vi "robot_dis.vi"() -> ()   [LabVIEW 2014]
uses:
  <vilib>/robotics/Controls/2D Rangefinder/NI_Robotics_2D Rangefinder.xctl
  <vilib>/Utility/error.llb/DialogType.ctl
  <vilib>/picture/3D Picture Control/Object/Create Object (drawable).vi
  <vilib>/picture/3D Picture Control/Object/Add Object (reference).vi
  <vilib>/picture/3D Picture Control/NI_3D Picture Control.lvlib
panel:
  out "布尔 3":bool=TRUE
  out "Lidar_two":i32
  out "StopChannelRecord":bool
  out "StartChannelRecord":bool
  out "布尔 2":bool
  in  "开始录像":bool
  in  "布尔":bool
  out "StartChannelRealPlay":bool
  in  "Lidar_data":cluster{"数组":dbl[], "数组 2":dbl[][]}
  out "Rangefinder Indicator":cluster{"angle":dbl[], "distance":dbl[][]}(xcontrol)
  out "扫描质量":u8
  out "Lidar_size":u16
  in  "distance":dbl[](array[numeric])
  in  "angle":dbl[](array[numeric])
  out "数值 2":u8 format="%x"
  out "x或y?":u8 format="%x"
  out "x = y?":bool
  out "无符号字节数组 2":u8[](array[numeric])
  out "动力电池":dbl(slide) scale=0.0..100.0
  out "控制电池":dbl(slide) scale=0.0..100.0 scale format="%.3f"
  in  "主要":refnum<k7>(container)
  in  "后摄像头":refnum<k7>(container)
  out "Login 2":i32
  out "前摄像头":bool
  out "后摄像头":bool
  out "Login":i32
  in  "前摄像头":refnum<k7>(container)
  in  "AUTO":bool
  in  "减速":bool
  in  "加速":bool
  in  "左":bool
  in  "右":bool
  in  "下":bool
  in  "上":bool
  in  "LED8":u8(slide) step=1 scale=0.0..100.0
  in  "LED7":u8(slide) step=1 scale=0.0..100.0
  in  "LED6":u8(slide) step=1 scale=0.0..100.0
  in  "LED5":u8(slide) step=1 scale=0.0..100.0
  in  "LED4":u8(slide) step=1 scale=0.0..100.0
  in  "LED3":u8(slide) step=1 scale=0.0..100.0
  in  "LED2":u8(slide) step=1 scale=0.0..100.0
  in  "LED1":u8(slide) step=1 scale=0.0..100.0
  in  "上下移动":dbl(slide) scale=-10.0..10.0
  in  "左右移动":dbl(slide) scale=-10.0..10.0
  in  "前后移动":dbl(slide) scale=-10.0..10.0
  in  "缩放":dbl(knob)=2.2771854734286614 scale=0.0..10.0
  out "小车方向":refnum<vi>(3d-picture)
  out "HEANDING":i32
  out "BANK":i32
  out "PITCH":i32
  in  "方向枚举":enum16{"停", "上", "下", "左", "右"}(ring)
  out "和":u8
  out "Car_lock":u8
  out "当前速度":u16
  out "当前方向":u8
  out "数据传输":bool
  in  "数据输入":string
  in  "QUIT":bool
  in  "WRITE":bool
  # "TETRAELC--机器人测试平台V0.1"
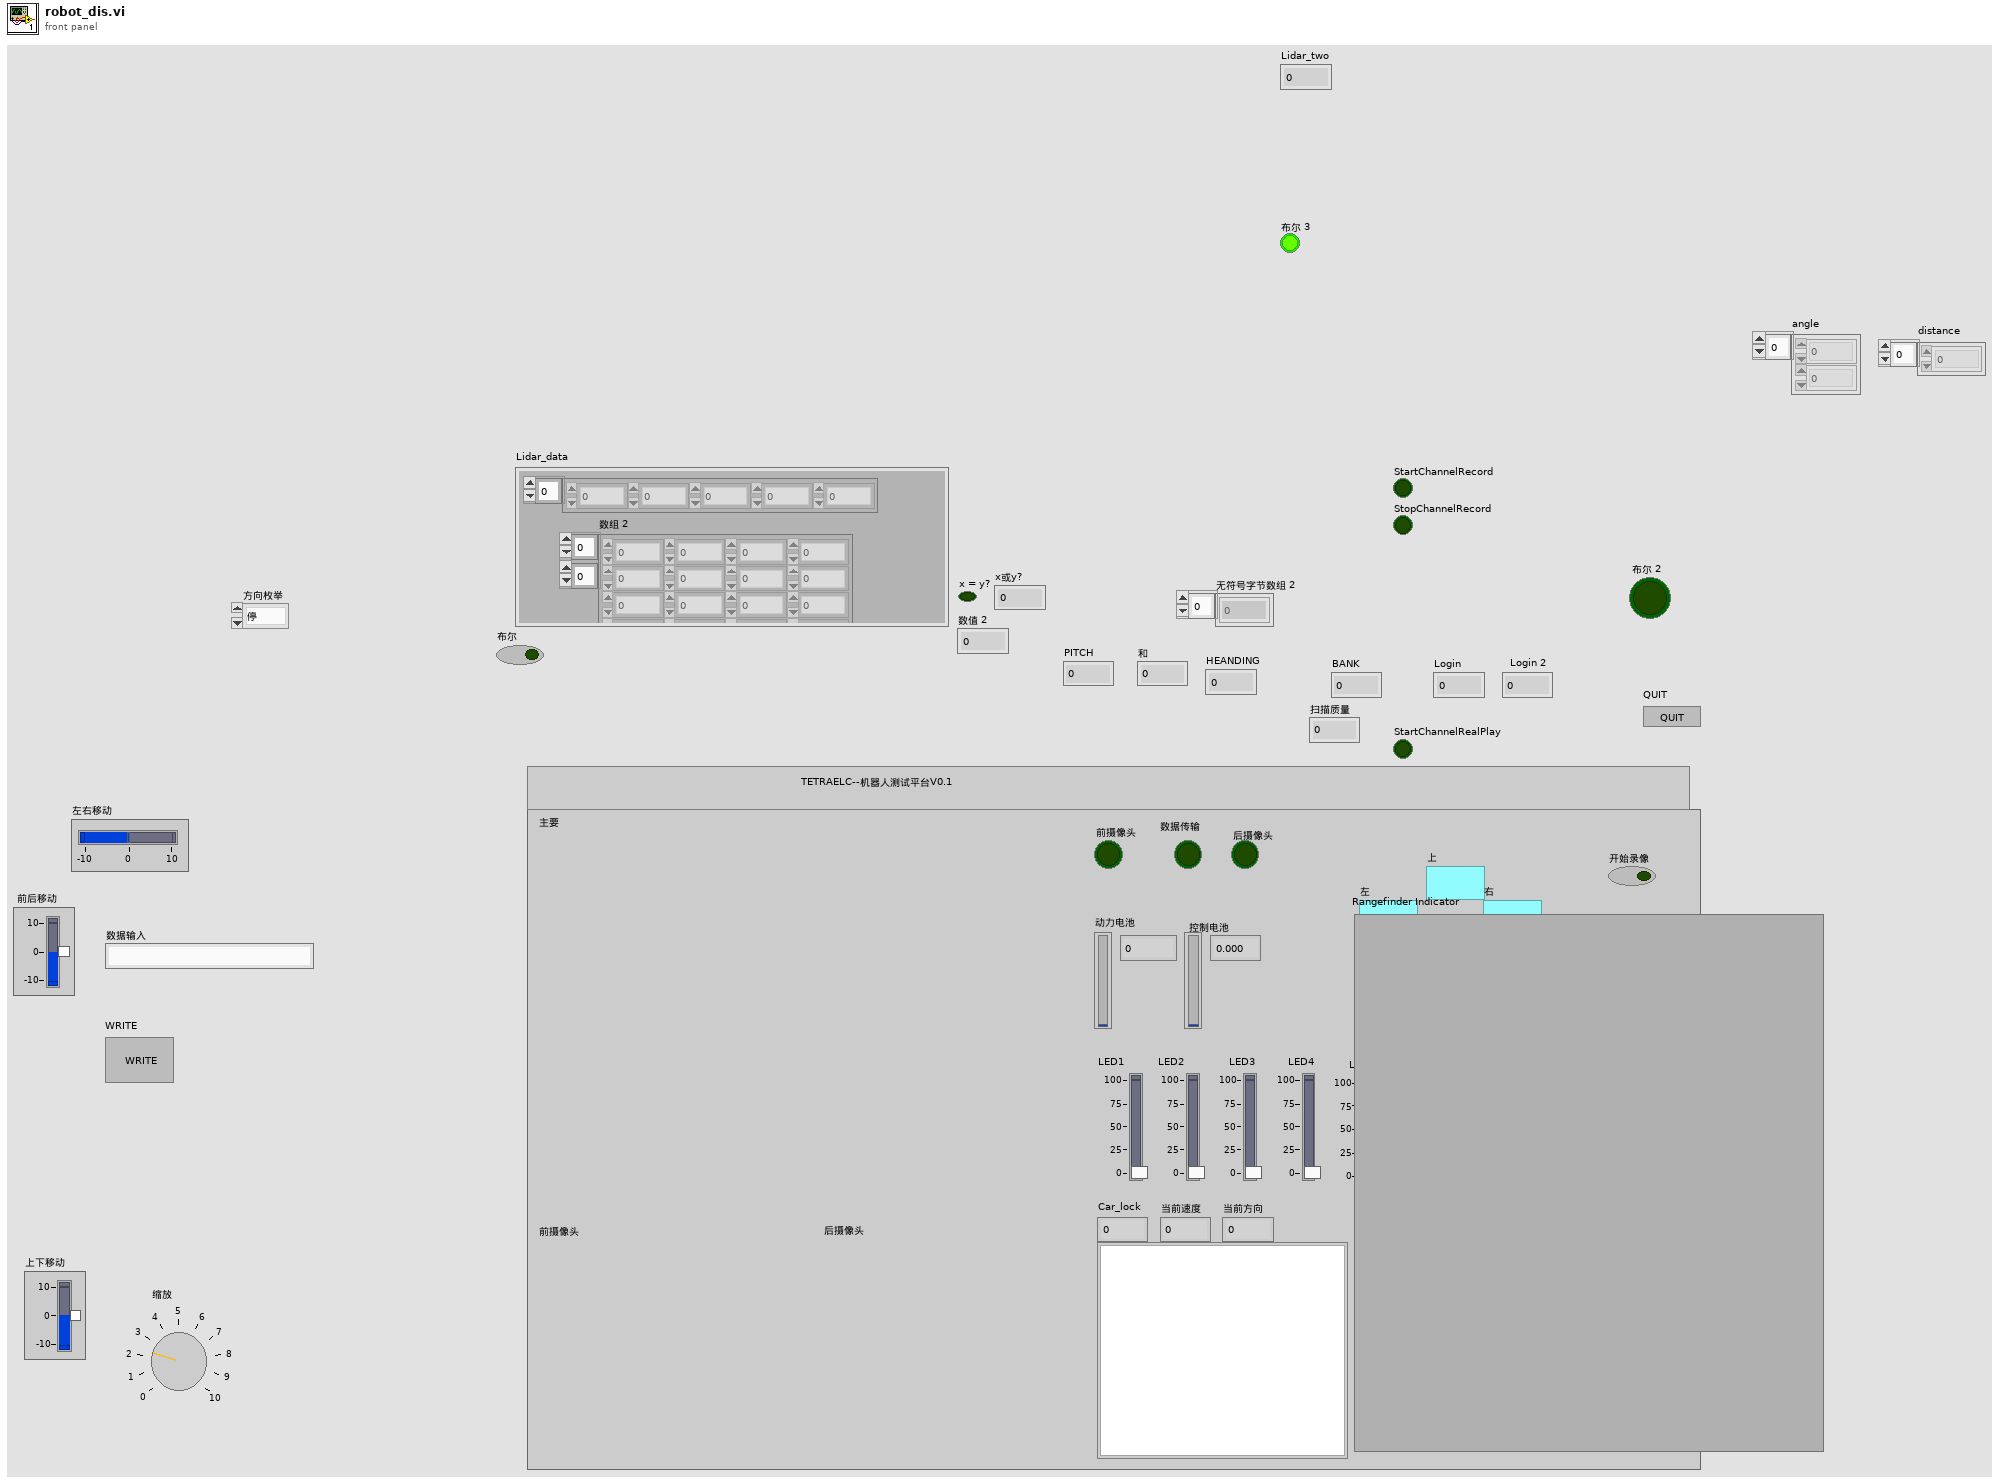
[diagram p1: front panel]
types:
  T1 = typedef "DialogType.ctl" = u16
  T2 = cluster{"PITCH":i32, "BANK":i32, "HEANDING":i32, "X":i32, "Y":i32, "Z":i32}
  T3 = cluster{"quality":u8, "angle":u16, "distance\n":u16}
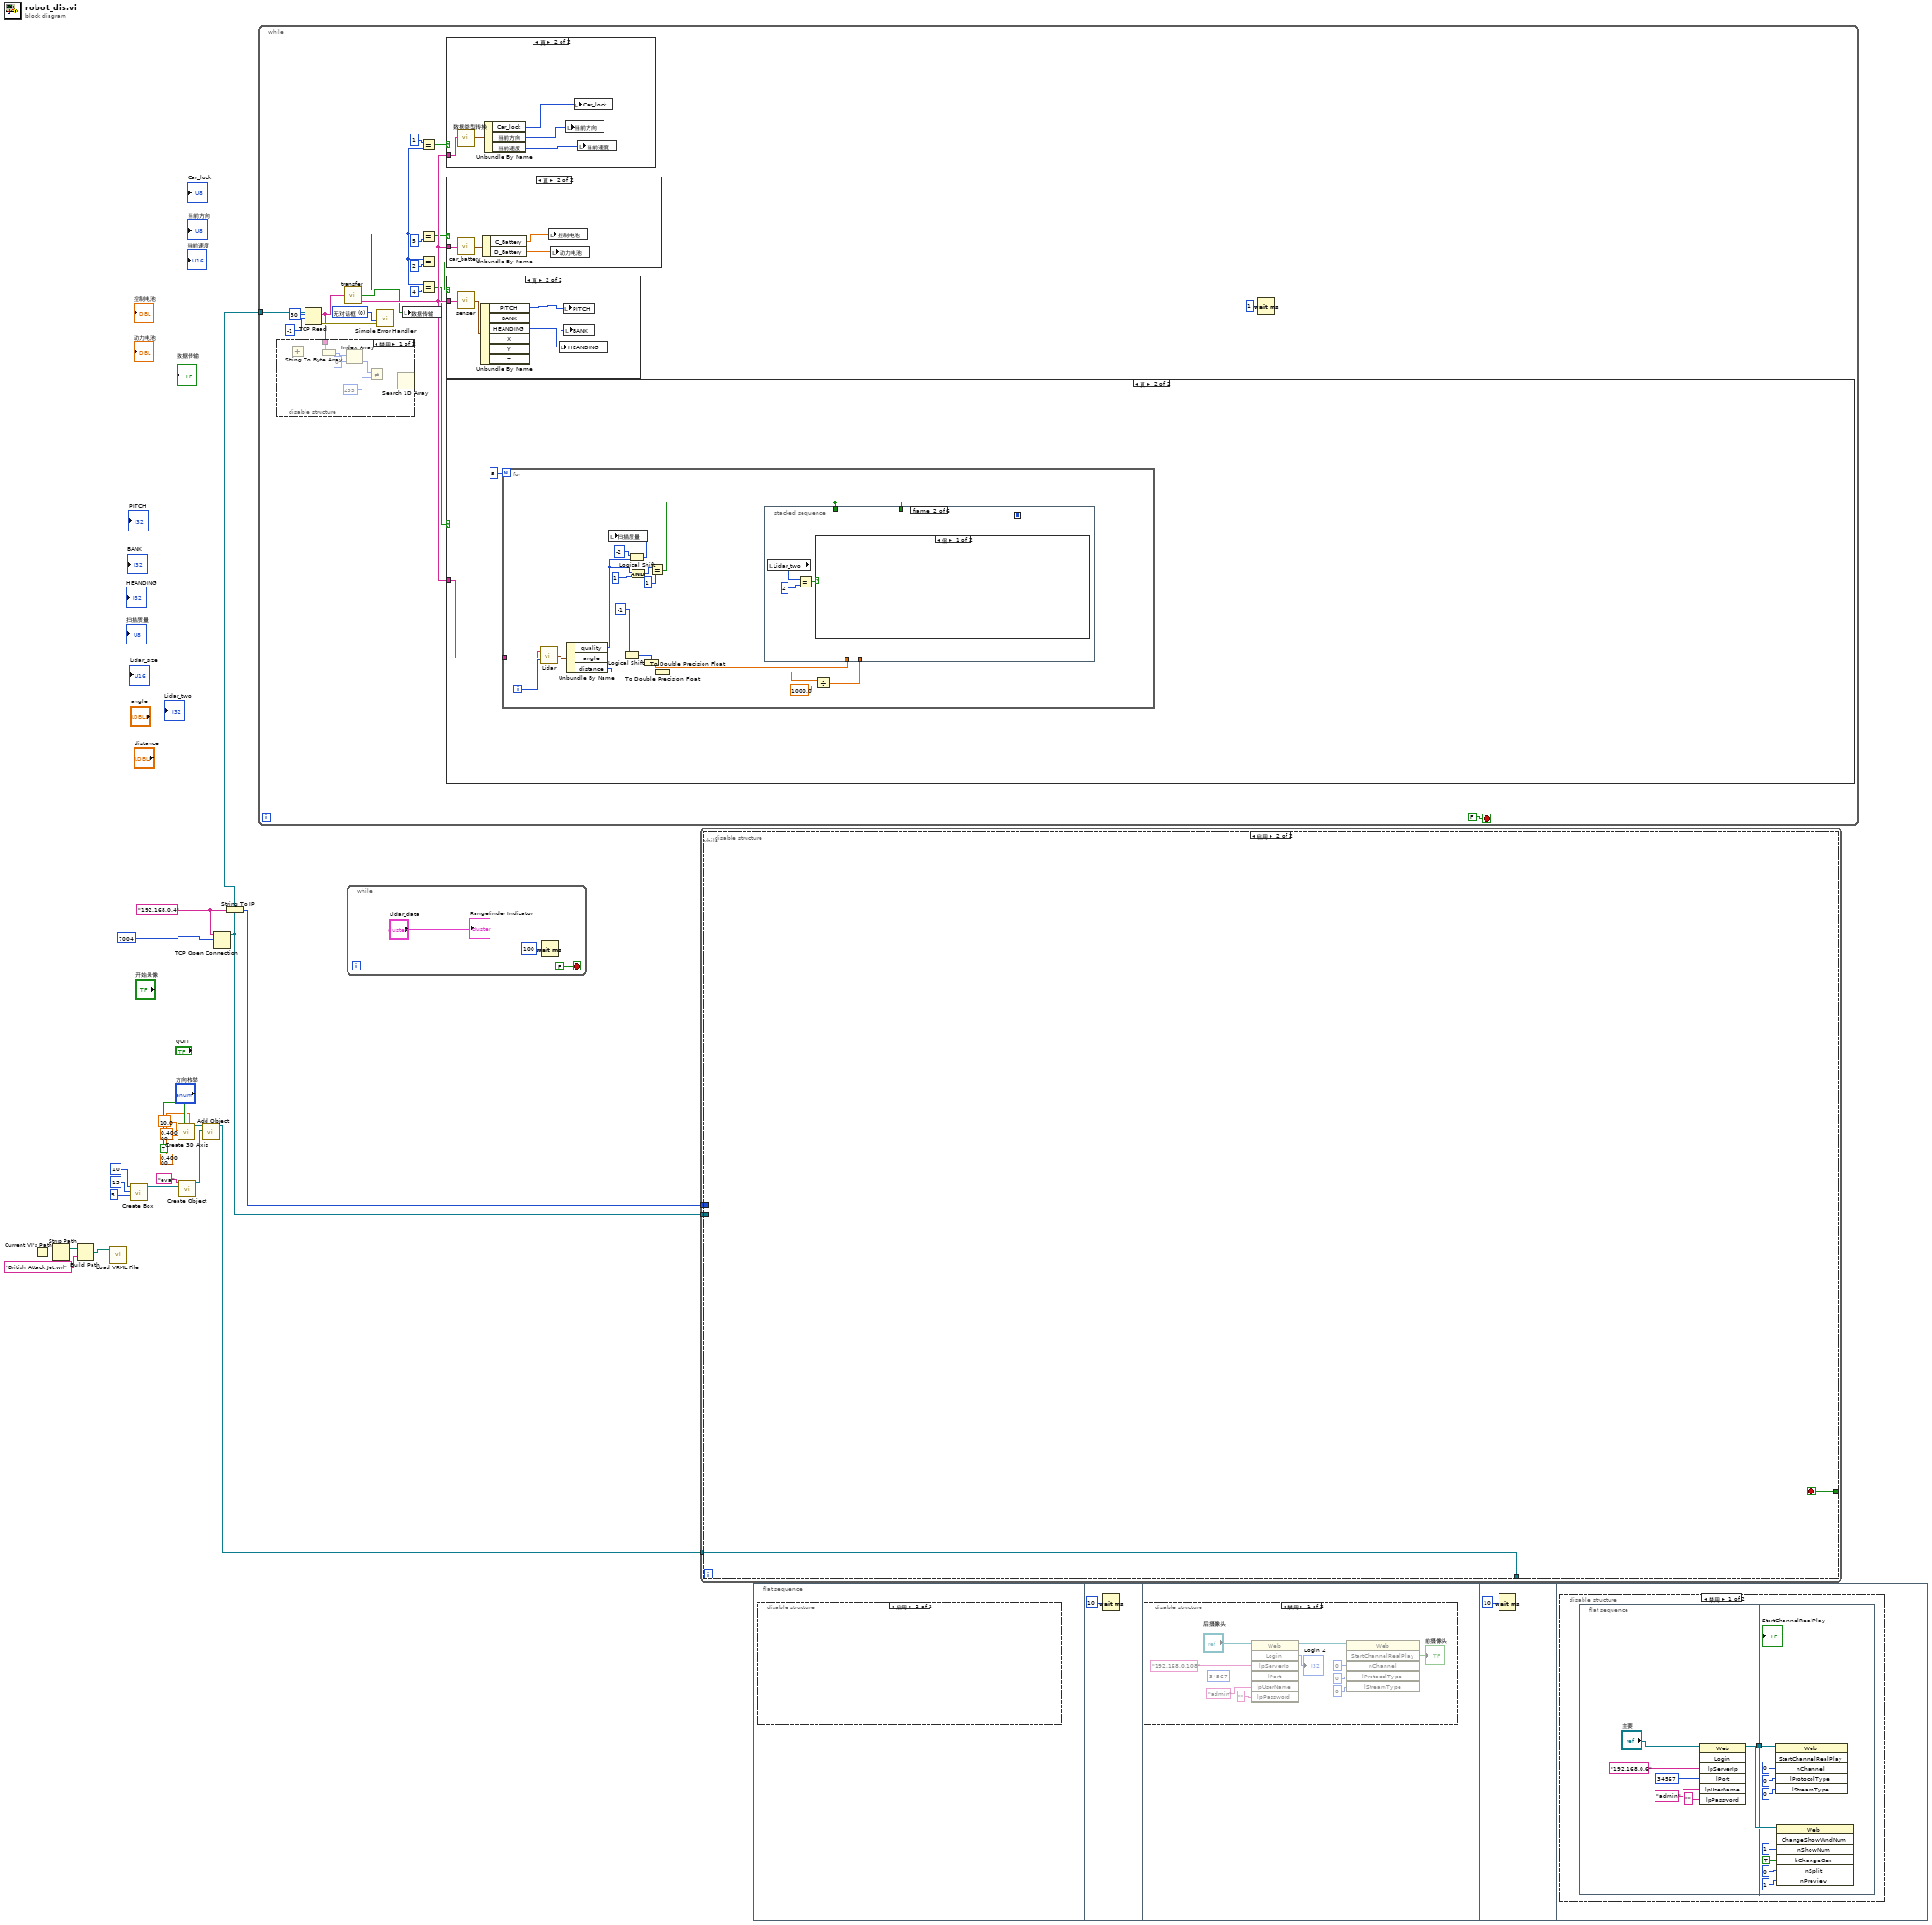
[diagram p0: block diagram]
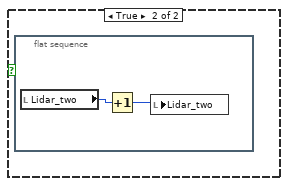
[diagram p5: hidden frame]
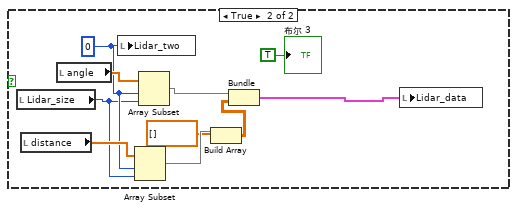
[diagram p6: hidden frame]
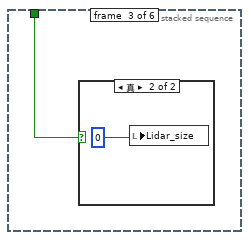
[diagram p7: hidden frame]
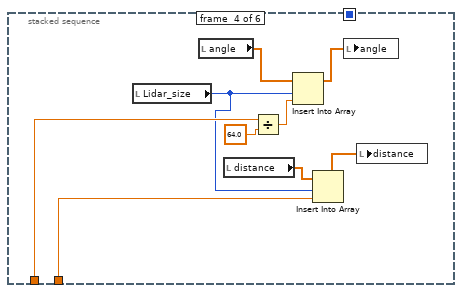
[diagram p9: hidden frame]
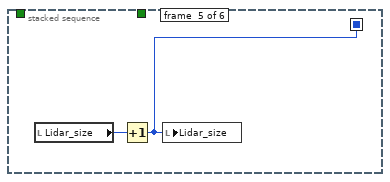
[diagram p10: hidden frame]
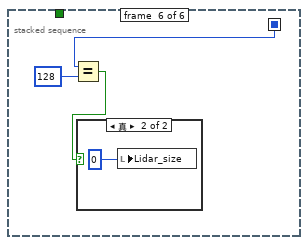
[diagram p11: hidden frame]
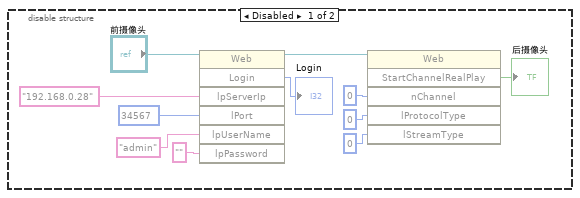
[diagram p16: hidden frame]
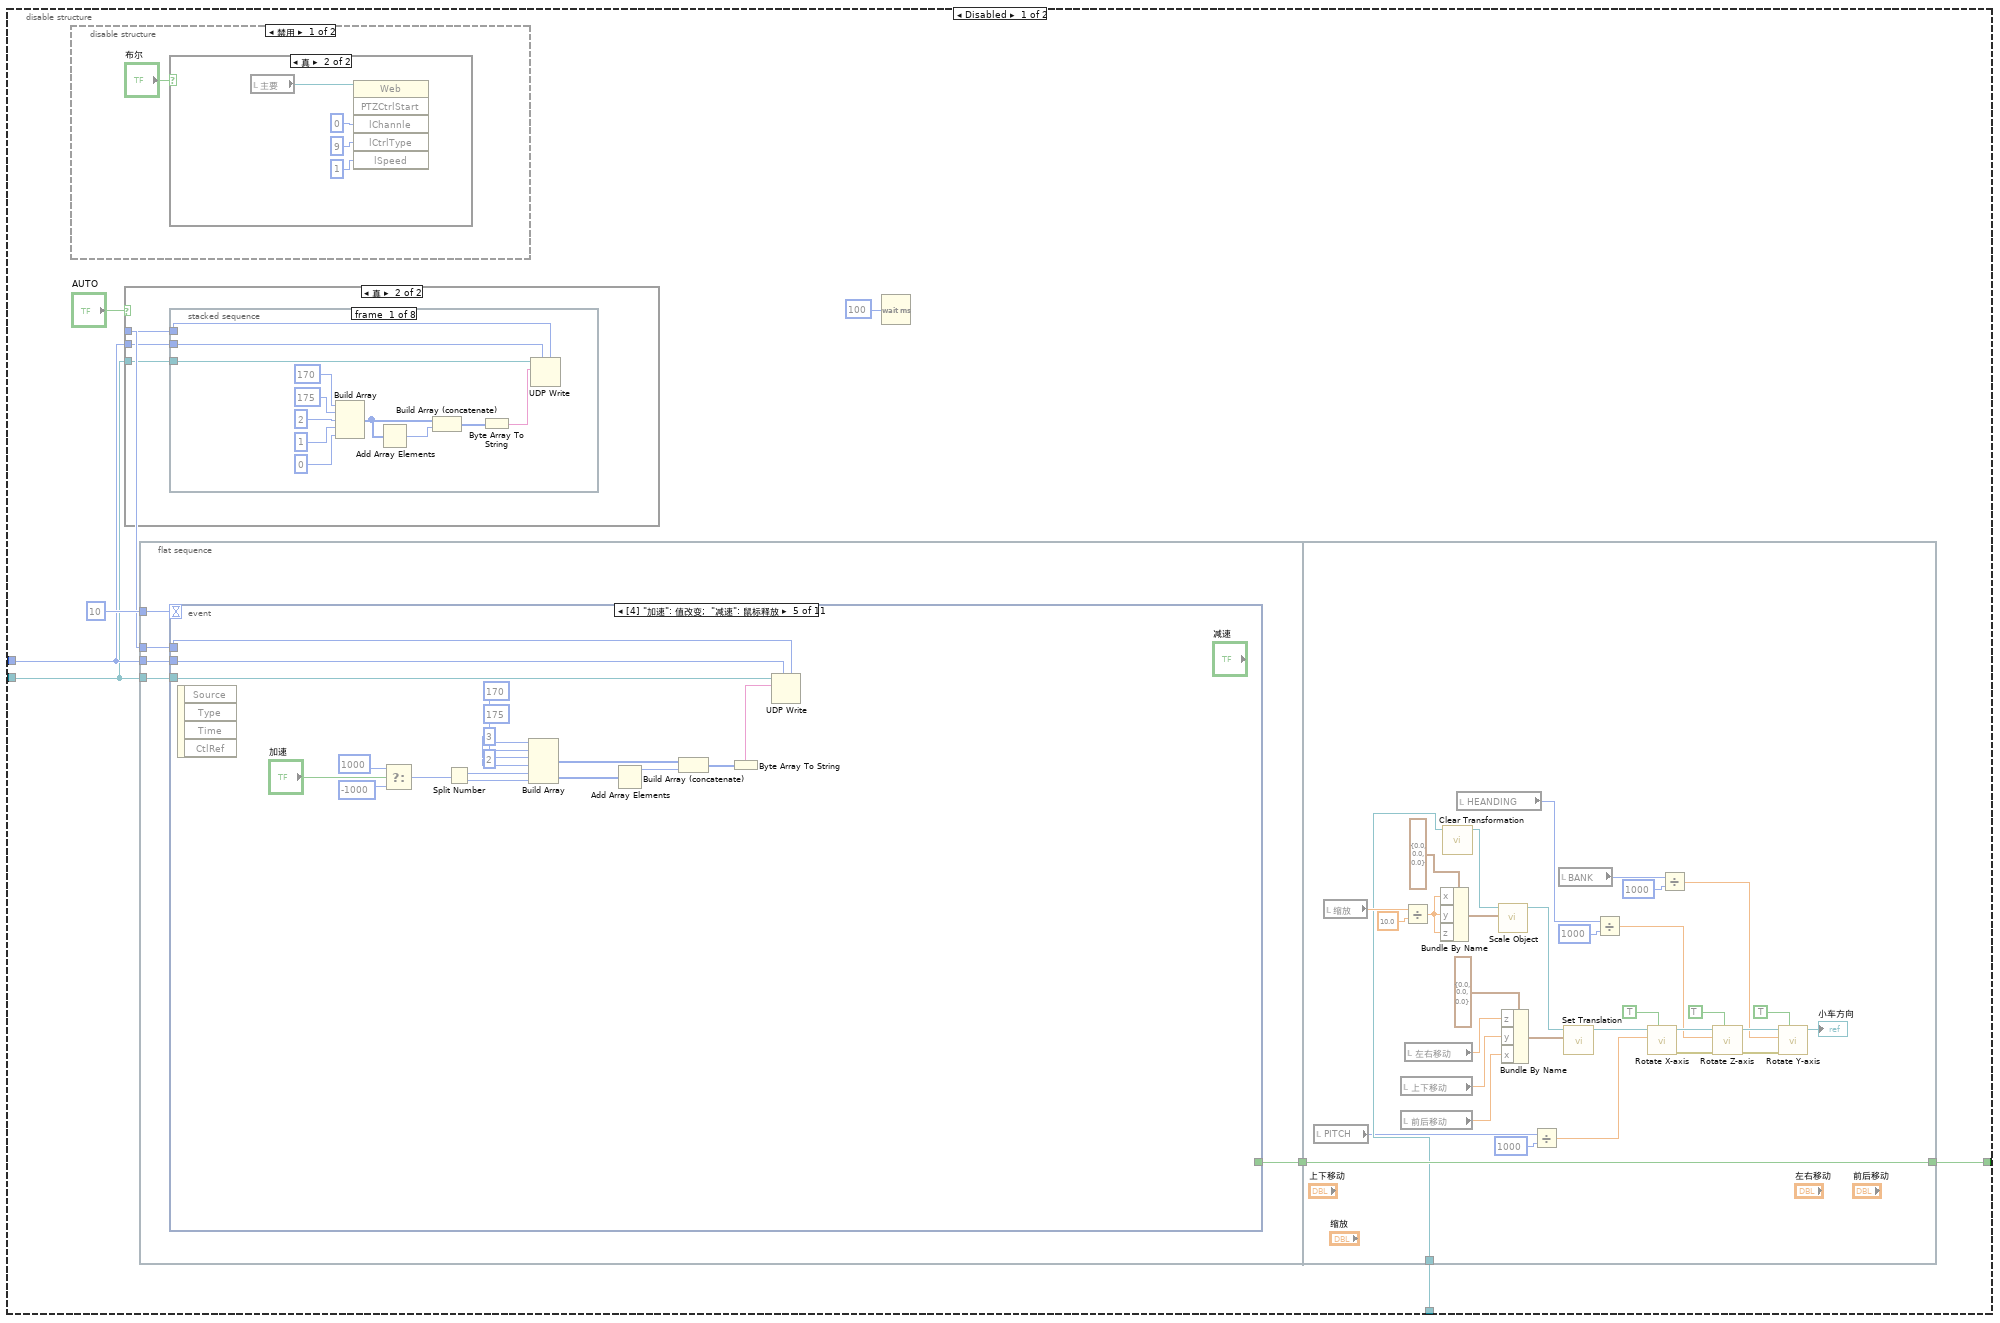
[diagram p19: hidden frame]
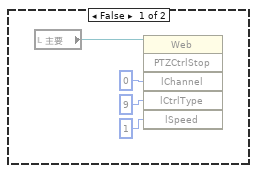
[diagram p20: hidden frame]
diagram:
  w1 = "192.168.0.4" ("目标主机")
  n1 = Current VI's Path() -> (path=w7:path)
  n2 = Strip Path(path=w7) -> (stripped path=w6:path)  [unwired: 1 out]
  n3 = Build Path(base path=w6, name or relative path="British Attack Jet.wrl" ("Name")) -> (appended path=w8:path)
  n4 = call <vilib>:"Load VRML File.vi"("Path"=w8) -> ()  [unwired: 9 in, 2 out]
  n5 = call <vilib>:"Create Box.vi"("Length Z"=5, "Length Y"=15, "Length X"=10) -> ("New Box Refnum"=w15:refnum<vi>)  [unwired: 7 in, 1 out]
  n6 = call <vilib>:"Create 3D Axis.vi"("Character Size"=sgl 0.4, "Axis label?"=TRUE, "Radius"=sgl 0.4, "Length"=sgl 10.0) -> ("New Object Refnum"=w10:refnum<vi>)  [unwired: 6 in, 1 out]
  n7 = call-poly <vilib>:"Create Object.vi"("Geometry"=w15, "Name"="eva") -> ("Scene:New Object"=w4:refnum<vi>)  [unwired: 8 in, 1 out]
  n8 = call-poly <vilib>:"Add Object.vi"("New Object In"=w4, "Scene Object In"=w10) -> ("Scene Object Out"=w9:refnum<vi>)  [unwired: 7 in, 2 out]
  n9 = TCP Open Connection(address=w1, remote port or service name=u16 7004 ("本地端口")) -> (connection ID=w2:refnum<k5>)  [unwired: 3 in, 1 out]
  n10 = String To IP(1:w1) -> (0:w20:u32)
  n11 = while {
    tunnel: w2 -> [w25]
    stop <- FALSE stop-if-true
    w28 = T1 0 items=["无对话框", "确定信息", "继续或停止信息", "确定信息＋警告", "继续/停止+警告"] ("type of dialog (OK msg:1)")
    n12 = TCP Read(connection ID=w25, bytes to read=30 ("读取的字节"), 9:-1 ("超时毫秒(25000)")) -> (data out=w22:string, error out=w23:errorcluster)  [unwired: 2 in, 1 out]
    n13 = disable-structure shown="禁用" {
      disable-tunnel: w22 -> [w44 _]
      frame Disabled {
        n14 = Add() -> ()  [unwired: 2 in, 1 out]
        n15 = String To Byte Array(string=w44) -> (unsigned byte array=w43:u8[])
        n16 = Index Array(array=w43, index=0 ("索引")) -> (element=w41:u8)
        n17 = Not Equal?(x=w41, y=u8 255 ("元素")) -> ()  [unwired: 1 out]
        n18 = Search 1D Array() -> ()  [unwired: 3 in, 1 out]
      }
      frame Enabled {
      }
    }
    n19 = call "transfer.vi"("输入"=w22) -> ("数值"=w35:u8, "布尔"=w27:bool, "输出"=w38:string)
    n20 = call <vilib>:"Simple Error Handler.vi"("type of dialog (OK msg:1)"=w28, "error in (no error)"=w23) -> ()  [unwired: 3 in, 5 out]
    n21 = local write "数据传输"(w27) -> ()
    n22 = Equal?(x=u8 1, y=w35) -> (x = y?=w30:bool)
    n23 = Equal?(x=w35, y=u8 5 ("x")) -> (x = y?=w34:bool)
    n24 = Equal?(x=w35, y=u8 2 ("x")) -> (x = y?=w32:bool)
    n25 = Equal?(x=w35, y=u8 4 ("x")) -> (x = y?=w37:bool)
    n26 = case shown="真" w30 {
      tunnel: w38 -> [_ w107]
      frame False {
      }
      frame True {
        n27 = call "数据类型转换.vi"("read buffer"=w107) -> ("输出簇"=w106:cluster{"Car_lock":u8, "当前方向":u8, "当前速度\n":u16})
        n28 = Unbundle By Name(w106) -> ("Car_lock"=w105:u8, "当前方向"=w104:u8, "当前速度"=w103:u16)
        n29 = local write "当前方向"(w104) -> ()
        n30 = local write "Car_lock"(w105) -> ()
        n31 = local write "当前速度"(w103) -> ()
      }
    }
    n32 = case shown="真" w34 {
      tunnel: w38 -> [_ w111]
      frame False {
      }
      frame True {
        n33 = call "car_battery.vi"("read buffer"=w111) -> ("输出簇"=w110:cluster{"C_Battery":dbl, "D_Battery\n":dbl})
        n34 = Unbundle By Name(w110) -> ("C_Battery"=w109:dbl, "D_Battery"=w108:dbl)
        n35 = local write "控制电池"(w109) -> ()
        n36 = local write "动力电池"(w108) -> ()
      }
    }
    n37 = case shown="真" w32 {
      tunnel: w38 -> [_ w102]
      frame False {
      }
      frame True {
        n38 = call "senser.vi"("read buffer"=w102) -> ("输出簇"=w101:T2)
        n39 = Unbundle By Name(w101) -> ("PITCH"=w100:i32, "BANK"=w99:i32, "HEANDING"=w98:i32)  [unwired: 3 out]
        n40 = local write "HEANDING"(w98) -> ()
        n41 = local write "PITCH"(w100) -> ()
        n42 = local write "BANK"(w99) -> ()
      }
    }
    n43 = case shown="真" w37 {
      tunnel: w38 -> [_ w46]
      frame False {
      }
      frame True {
        n44 = for {
          N: 5 -> [_]
          tunnel: w46 -> [w49]
          i -> [w47]
          n45 = call "Lidar.vi"("数值"=w47, "read buffer"=w49) -> ("输出簇"=w48:T3)
          n46 = Unbundle By Name(w48) -> ("quality"=w57:u8, "angle"=w61:u16, "distance"=w53:u16)
          n47 = Logical Shift(y=i16 -1, x=w61) -> (x << y=w60:u16)
          n48 = Logical Shift(y=i16 -2, x=w57) -> (x << y=w62:u8)
          n49 = local write "扫描质量"(w62) -> ()
          n50 = And(x=w57, y=u8 1) -> (x .and. y?=w56:u8)
          n51 = To Double Precision Float(number=w60) -> (double precision float=w58:dbl)
          n52 = Equal?(x=w56, y=u8 1) -> (x = y?=w54:bool)
          n53 = To Double Precision Float(number=w53) -> (double precision float=w52:dbl)
          n54 = Divide(x=w52, y=1000.0) -> (x/y=w50:dbl)
          n55 = stacked-sequence {
            seq-local: [_ _ _ _ w92 _] -> [_ _ _ _ _ w95]
            tunnel: w54 -> [w65 _ _ _ _ _]
            tunnel: w54 -> [_ _ w81 _ _ _]
            tunnel: w58 -> [_ _ _ w88 _ _]
            tunnel: w50 -> [_ _ _ w83 _ _]
            frame #0 {
              n56 = case shown="假" w65 {
                frame False {
                }
                frame True {
                  n57 = flat-sequence {
                    frame #0 {
                      n58 = local read "Lidar_two"() -> (w67:i32)
                      n59 = Increment(x=w67) -> (x+1=w66:i32)
                      n60 = local write "Lidar_two"(w66) -> ()
                    }
                  }
                }
              }
            }
            frame #1 {
              n61 = local read "Lidar_two"() -> (w70:i32)
              n62 = Equal?(x=w70, y=2) -> (x = y?=w68:bool)
              n63 = case shown="假" w68 {
                frame False {
                }
                frame True {
                  w78 = 0 ("Lidar_two")
                  n64 = local read "Lidar_size"() -> (w77:u16)
                  n65 = local read "distance"() -> (w79:dbl[])
                  n66 = local read "angle"() -> (w80:dbl[])
                  n67 = local write "Lidar_two"(w78) -> ()
                  n68 = Array Subset(array=w79, index=w78, length=w77) -> (w76:dbl[])
                  n69 = Array Subset(array=w80, index=w78, length=w77) -> (w74:dbl[])
                  n70 = Build Array(w76, dbl[] [] ("元素")) -> (w73:dbl[][])
                  n71 = Bundle(w74, w73) -> (w71:cluster{dbl[], dbl[][]})  [unwired: 1 in]
                  n72 = local write "Lidar_data"(w71) -> ()
                  "布尔 3" <- TRUE
                }
              }
            }
            frame #2 {
              n73 = case shown="真" w81 {
                frame False {
                }
                frame True {
                  n74 = local write "Lidar_size"(u8 0 ("Lidar_size")) -> ()
                }
              }
            }
            frame #3 {
              n75 = local read "Lidar_size"() -> (w84:u16)
              n76 = local read "angle"() -> (w91:dbl[])
              n77 = local read "distance"() -> (w85:dbl[])
              n78 = Divide(x=w88, y=64.0) -> (x/y=w87:dbl)
              n79 = Insert Into Array(array=w91, index=w84, new element=w87) -> (w90:dbl[])
              n80 = Insert Into Array(array=w85, index=w84, new element=w83) -> (w86:dbl[])
              n81 = local write "angle"(w90) -> ()
              n82 = local write "distance"(w86) -> ()
            }
            frame #4 {
              n83 = local read "Lidar_size"() -> (w93:u16)
              n84 = Increment(x=w93) -> (x+1=w92:u16)
              n85 = local write "Lidar_size"(w92) -> ()
            }
            frame #5 {
              n86 = Equal?(x=w95, y=u16 128) -> (x = y?=w94:bool)
              n87 = case shown="真" w94 {
                frame False {
                }
                frame True {
                  n88 = local write "Lidar_size"(u16 0 ("Lidar_size")) -> ()
                }
              }
            }
          }
        }
      }
    }
    n89 = Wait (ms)(milliseconds to wait=u32 1 ("等待时间（毫秒）")) -> ()  [unwired: 1 out]
  }
  n90 = while {
    stop <- FALSE stop-if-true
    n91 = Wait (ms)(milliseconds to wait=u32 100 ("等待时间（毫秒）")) -> ()  [unwired: 1 out]
    "Rangefinder Indicator" <- "Lidar_data"
  }
  n92 = while {
    tunnel: w2 -> [w115]
    tunnel: w20 -> [w116]
    tunnel: w9 -> [w117]
    stop <- w118 stop-if-true
    n93 = disable-structure shown="启用" {
      disable-tunnel: [w126 _] -> w118
      disable-tunnel: w117 -> [w124 _]
      disable-tunnel: w116 -> [w122 _]
      disable-tunnel: w115 -> [w121 _]
      frame Disabled {
        n94 = disable-structure shown="禁用" {
          frame Disabled {
            n95 = case shown="真" "布尔" {
              frame False {
                n96 = local read "主要"() -> (w132:refnum<k7>)
                n97 = invoke class="Web" method="PTZCtrlStop"(reference=w132, "lChannel"=0, "lCtrlType"=9, "lSpeed"=1) -> ()  [unwired: 2 in, 6 out]
              }
              frame True {
                n98 = local read "主要"() -> (w136:refnum<k7>)
                n99 = invoke class="Web" method="PTZCtrlStart"(reference=w136, "lChannle"=0, "lCtrlType"=9, "lSpeed"=1) -> ()  [unwired: 2 in, 6 out]
              }
            }
          }
          frame Enabled {
          }
        }
        n100 = case shown="真" "AUTO" {
          tunnel: [_ w139] -> w123
          tunnel: w122 -> [_ w138]
          tunnel: w121 -> [_ w137]
          frame False {
          }
          frame True {
            n101 = stacked-sequence {
              tunnel: w139 -> [w142 _ w153 _ w167 _ w180 _]
              tunnel: w138 -> [w141 _ w154 _ w168 _ w181 _]
              tunnel: w137 -> [w140 _ w155 _ w169 _ w179 _]
              frame #0 {
                n102 = Build Array(u8 170 ("元素"), u8 175 ("元素"), u8 2 ("元素"), u8 1 ("元素"), u8 0 ("元素")) -> (w146:u8[])
                n103 = Add Array Elements(numeric array=w146) -> (sum=w145:u8)
                n104 = Build Array (concatenate)(w146, w145) -> (w144:u8[])
                n105 = Byte Array To String(unsigned byte array=w144) -> (string=w151:string)
                n106 = UDP Write(address=w141, port or service name=w142, connection ID=w140, data in=w151) -> ()  [unwired: 2 in, 2 out]
              }
              frame #1 {
                n107 = Wait (ms)(milliseconds to wait=u32 3000 ("等待时间（毫秒）")) -> ()  [unwired: 1 out]
              }
              frame #2 {
                n108 = Build Array(u8 170 ("元素"), u8 175 ("元素"), u8 2 ("元素"), u8 1 ("元素"), u8 8 ("元素")) -> (w159:u8[])
                n109 = Add Array Elements(numeric array=w159) -> (sum=w158:u8)
                n110 = Build Array (concatenate)(w159, w158) -> (w157:u8[])
                n111 = Byte Array To String(unsigned byte array=w157) -> (string=w164:string)
                n112 = UDP Write(address=w154, port or service name=w153, connection ID=w155, data in=w164) -> ()  [unwired: 2 in, 2 out]
              }
              frame #3 {
                n113 = Wait (ms)(milliseconds to wait=u32 1000 ("等待时间（毫秒）")) -> ()  [unwired: 1 out]
              }
              frame #4 {
                n114 = Build Array(u8 170 ("元素"), u8 175 ("元素"), u8 2 ("元素"), u8 1 ("元素"), u8 1 ("元素")) -> (w173:u8[])
                n115 = Add Array Elements(numeric array=w173) -> (sum=w172:u8)
                n116 = Build Array (concatenate)(w173, w172) -> (w171:u8[])
                n117 = Byte Array To String(unsigned byte array=w171) -> (string=w177:string)
                n118 = UDP Write(address=w168, port or service name=w167, connection ID=w169, data in=w177) -> ()  [unwired: 2 in, 2 out]
              }
              frame #5 {
                n119 = Wait (ms)(milliseconds to wait=u32 3000 ("等待时间（毫秒）")) -> ()  [unwired: 1 out]
              }
              frame #6 {
                n120 = Build Array(u8 170 ("元素"), u8 175 ("元素"), u8 2 ("元素"), u8 1 ("元素"), u8 8 ("元素")) -> (w185:u8[])
                n121 = Add Array Elements(numeric array=w185) -> (sum=w184:u8)
                n122 = Build Array (concatenate)(w185, w184) -> (w183:u8[])
                n123 = Byte Array To String(unsigned byte array=w183) -> (string=w190:string)
                n124 = UDP Write(address=w181, port or service name=w180, connection ID=w179, data in=w190) -> ()  [unwired: 2 in, 2 out]
              }
              frame #7 {
                n125 = Wait (ms)(milliseconds to wait=u32 1000 ("等待时间（毫秒）")) -> ()  [unwired: 1 out]
              }
            }
          }
        }
        n126 = flat-sequence {
          tunnel: [w196] -> w127
          tunnel: 10 -> [w195]
          tunnel: w121 -> [w194]
          tunnel: w122 -> [w193]
          tunnel: w123 -> [w192]
          tunnel: [w415] -> w126
          tunnel: w127 -> [w415]
          tunnel: w124 -> [w389]
          frame #0 {
            n127 = event shown="[4] \"加速\": 值改变;  \"减速\": 鼠标释放" {
              selector: _ -> [_ _ _ _ _ _ _ _ _ _ _]
              dyn-events: _ -> [_ _ _ _ _ _ _ _ _ _ _]
              timeout: w195 -> [_ _ _ _ _ _ _ _ _ _ _]
              tunnel: [_ _ _ _ _ _ _ _ _ _ TRUE] -> w196
              tunnel: w194 -> [_ _ _ w259 w276 w296 w309 w331 w353 w378 w382]
              tunnel: w193 -> [_ _ _ w260 w277 w297 w310 w332 w354 w377 _]
              tunnel: w192 -> [_ _ _ w261 w278 w298 w311 w333 w355 w376 _]
              event Timeout {
                n128 = event-data() -> ()  [unwired: 1 in, 1 out]
                n129 = disable-structure shown="启用" {
                  disable-tunnel: _ -> [w213 _]
                  frame Disabled {
                    n130 = String Subset(string=w213, offset (0)=0 ("长度（剩余）"), length (rest)=100 ("长度（剩余）")) -> (substring=w223:string)
                    n131 = String To Byte Array(string=w223) -> (unsigned byte array=w210:u8[])
                    "无符号字节数组 2" <- w210
                    n132 = Index Array(array=w210, index #1=0 ("索引"), index #2=1 ("索引")) -> (element #1=w201:u8, element #2=w200:u8)
                    n133 = for {
                      N: 83 -> [_]
                      tunnel: w210 -> [w230]
                      shift-right: [w225] -> w199
                      shift-left: _ -> [w224]
                      i -> [w229]
                      n134 = Add(x=2, y=w229) -> (x+y=w227:i32)
                      n135 = Index Array(array=w230, index=w227) -> (element=w226:u8)
                      n136 = Exclusive Or(1:w224, 2:w226) -> (0:w225:u8)
                    }
                    "数值 2" <- w199
                    n137 = And(x=w200, y=u8 15) -> (x .and. y?=w203:u8)
                    n138 = Logical Shift(y=i16 -4, x=w201) -> (x << y=w216:u8)
                    n139 = Logical Shift(y=i16 -4, x=w200) -> (x << y=w214:u8)
                    n140 = Equal?(x=w214, y=u8 5) -> (x = y?=w211:bool)
                    n141 = Logical Shift(y=i16 4, x=w203) -> (x << y=w205:u8)
                    n142 = And(x=w201, y=u8 15) -> (x .and. y?=w204:u8)
                    n143 = Equal?(x=w216, y=u8 10) -> (x = y?=w212:bool)
                    n144 = And(x=w212, y=w211) -> (x .and. y?=w197:bool)
                    n145 = Or(x=w205, y=w204) -> (x .or. y?=w198:u8)
                    "x或y?" <- w198
                    n146 = case shown="真" w197 {
                      frame False {
                      }
                      frame True {
                        n147 = while {
                          stop <- FALSE stop-if-true
                        }
                        n148 = local read item#-1() -> (w232)
                        n149 = Increment(x=w232) -> (x+1=w231:dbl)
                        n150 = local write item#-1(w231) -> ()
                      }
                    }
                    n151 = Equal?(x=w198, y=w199) -> ()  [unwired: 1 out]
                  }
                  frame Enabled {
                  }
                }
              }
              event "Lidar_two": Value Change {
                n152 = event-data() -> ()  [unwired: 1 in, 6 out]
                n153 = disable-structure shown="禁用" {
                  frame Disabled {
                    n154 = local read "Lidar_two"() -> (w236:i32)
                    n155 = Equal?(x=w236, y=2) -> (x = y?=w234:bool)
                    n156 = case shown="真" w234 {
                      frame False {
                      }
                      frame True {
                      }
                    }
                  }
                  frame Enabled {
                  }
                }
              }
              event "开始录像": Value Change {
                n157 = event-data() -> ()  [unwired: 1 in, 6 out]
                n158 = local read "开始录像"() -> (w238:bool)
                n159 = local read "主要"() -> (w239:refnum<k7>)
                n160 = case shown="真" w238 {
                  tunnel: w239 -> [w243 w248]
                  tunnel: [FALSE ("布尔 2") TRUE ("布尔 2")] -> w237
                  frame False {
                    n161 = invoke class="Web" method="StopChannelRecord"(reference=w243, "nChannel"=0) -> ("StopChannelRecord"=→"StopChannelRecord":bool)  [unwired: 2 in, 3 out]
                  }
                  frame True {
                    n162 = invoke class="Web" method="StartChannelRecord"(reference=w248, "nChannel"=0, "lpSaveFile"="D:\\record", "nType"=0) -> ("StartChannelRecord"=→"StartChannelRecord":bool)  [unwired: 2 in, 5 out]
                  }
                }
                "布尔 2" <- w237
              }
              event "LED1", "LED2", "LED3", "LED4", "LED5", "LED6", "LED7", "LED8": Value Change {
                n163 = event-data() -> ()  [unwired: 1 in, 6 out]
                n164 = Build Array(u8 170 ("元素"), u8 175 ("元素"), u8 4 ("元素"), u8 8 ("元素"), "LED1", "LED2", "LED3", "LED4", "LED5", "LED6", "LED7", "LED8") -> (w265:u8[])
                n165 = Add Array Elements(numeric array=w265) -> (sum=w264:u8)
                "和" <- w264
                n166 = Build Array (concatenate)(w265, w264) -> (w263:u8[])
                n167 = Byte Array To String(unsigned byte array=w263) -> (string=w258:string)
                n168 = UDP Write(address=w260, port or service name=w261, connection ID=w259, data in=w258, 9:250 ("超时毫秒(25000)")) -> ()  [unwired: 1 in, 2 out]
              }
              event "加速": Value Change; "减速": Mouse Up {
                n169 = event-data() -> ()  [unwired: 1 in, 4 out]
                n170 = Select(t=i16 1000 ("x"), s="加速", f=i16 -1000) -> (s? t:f=w271:i16)
                n171 = Split Number(x=w271) -> (hi(x)=w275:u8, lo(x)=w274:u8)
                n172 = Build Array(u8 170 ("元素"), u8 175 ("元素"), u8 3 ("元素"), u8 2 ("元素"), w275, w274) -> (w281:u8[])
                n173 = Add Array Elements(numeric array=w281) -> (sum=w280:u8)
                n174 = Build Array (concatenate)(w281, w280) -> (w279:u8[])
                n175 = Byte Array To String(unsigned byte array=w279) -> (string=w286:string)
                n176 = UDP Write(address=w277, port or service name=w278, connection ID=w276, data in=w286) -> ()  [unwired: 2 in, 2 out]
              }
              event "上": Value Change {
                n177 = event-data() -> ()  [unwired: 1 in, 6 out]
                n178 = flat-sequence {
                  tunnel: [w303] -> w287
                  frame #0 {
                    n179 = case shown="真" "上" {
                      frame False {
                        n180 = local write "方向枚举"(enum16{"停", "上", "下", "左", "右"}."停") -> ()
                      }
                      frame True {
                        n181 = local write "方向枚举"(enum16{"停", "上", "下", "左", "右"}."上") -> ()
                      }
                    }
                  }
                  frame #1 {
                    n182 = local read "方向枚举"() -> (w302:enum16{"停", "上", "下", "左", "右"})
                    n183 = case shown="\"上\", 默认" w302 {
                      tunnel: [u8 0 ("元素") u8 1 ("元素") u8 2 ("元素") u8 3 ("元素") u8 8 ("元素")] -> w303
                      frame "上", Default {
                      }
                      frame "下" {
                      }
                      frame "左" {
                      }
                      frame "右" {
                      }
                      frame "停" {
                      }
                    }
                  }
                }
                n184 = Build Array(u8 170 ("元素"), u8 175 ("元素"), u8 2 ("元素"), u8 1 ("元素"), w287) -> (w290:u8[])
                n185 = Add Array Elements(numeric array=w290) -> (sum=w289:u8)
                n186 = Build Array (concatenate)(w290, w289) -> (w288:u8[])
                n187 = Byte Array To String(unsigned byte array=w288) -> (string=w295:string)
                n188 = UDP Write(address=w297, port or service name=w298, connection ID=w296, data in=w295) -> ()  [unwired: 2 in, 2 out]
              }
              event "下": Value Change {
                n189 = event-data() -> ()  [unwired: 1 in, 6 out]
                n190 = flat-sequence {
                  tunnel: [w325] -> w312
                  frame #0 {
                    n191 = case shown="真" "下" {
                      frame False {
                        n192 = local write "方向枚举"(enum16{"停", "上", "下", "左", "右"}."停") -> ()
                      }
                      frame True {
                        n193 = local write "方向枚举"(enum16{"停", "上", "下", "左", "右"}."下") -> ()
                      }
                    }
                  }
                  frame #1 {
                    n194 = local read "方向枚举"() -> (w324:enum16{"停", "上", "下", "左", "右"})
                    n195 = case shown="\"上\", 默认" w324 {
                      tunnel: [u8 0 ("元素") u8 1 ("元素") u8 2 ("元素") u8 3 ("元素") u8 8 ("元素")] -> w325
                      frame "上", Default {
                      }
                      frame "下" {
                      }
                      frame "左" {
                      }
                      frame "右" {
                      }
                      frame "停" {
                      }
                    }
                  }
                }
                n196 = Build Array(u8 170 ("元素"), u8 175 ("元素"), u8 2 ("元素"), u8 1 ("元素"), w312) -> (w315:u8[])
                n197 = Add Array Elements(numeric array=w315) -> (sum=w314:u8)
                n198 = Build Array (concatenate)(w315, w314) -> (w313:u8[])
                n199 = Byte Array To String(unsigned byte array=w313) -> (string=w320:string)
                n200 = UDP Write(address=w310, port or service name=w311, connection ID=w309, data in=w320) -> ()  [unwired: 2 in, 2 out]
              }
              event "左": Value Change {
                n201 = event-data() -> ()  [unwired: 1 in, 6 out]
                n202 = flat-sequence {
                  tunnel: [w347] -> w334
                  frame #0 {
                    n203 = case shown="真" "左" {
                      frame False {
                        n204 = local write "方向枚举"(enum16{"停", "上", "下", "左", "右"}."停") -> ()
                      }
                      frame True {
                        n205 = local write "方向枚举"(enum16{"停", "上", "下", "左", "右"}."左") -> ()
                      }
                    }
                  }
                  frame #1 {
                    n206 = local read "方向枚举"() -> (w346:enum16{"停", "上", "下", "左", "右"})
                    n207 = case shown="\"上\", 默认" w346 {
                      tunnel: [u8 0 ("元素") u8 1 ("元素") u8 2 ("元素") u8 3 ("元素") u8 8 ("元素")] -> w347
                      frame "上", Default {
                      }
                      frame "下" {
                      }
                      frame "左" {
                      }
                      frame "右" {
                      }
                      frame "停" {
                      }
                    }
                  }
                }
                n208 = Build Array(u8 170 ("元素"), u8 175 ("元素"), u8 2 ("元素"), u8 1 ("元素"), w334) -> (w337:u8[])
                n209 = Add Array Elements(numeric array=w337) -> (sum=w336:u8)
                n210 = Build Array (concatenate)(w337, w336) -> (w335:u8[])
                n211 = Byte Array To String(unsigned byte array=w335) -> (string=w342:string)
                n212 = UDP Write(address=w332, port or service name=w333, connection ID=w331, data in=w342) -> ()  [unwired: 2 in, 2 out]
              }
              event "右": Value Change {
                n213 = event-data() -> ()  [unwired: 1 in, 6 out]
                n214 = flat-sequence {
                  tunnel: [w369] -> w356
                  frame #0 {
                    n215 = case shown="真" "右" {
                      frame False {
                        n216 = local write "方向枚举"(enum16{"停", "上", "下", "左", "右"}."停") -> ()
                      }
                      frame True {
                        n217 = local write "方向枚举"(enum16{"停", "上", "下", "左", "右"}."右") -> ()
                      }
                    }
                  }
                  frame #1 {
                    n218 = local read "方向枚举"() -> (w368:enum16{"停", "上", "下", "左", "右"})
                    n219 = case shown="\"上\", 默认" w368 {
                      tunnel: [u8 0 ("元素") u8 1 ("元素") u8 2 ("元素") u8 3 ("元素") u8 8 ("元素")] -> w369
                      frame "上", Default {
                      }
                      frame "下" {
                      }
                      frame "左" {
                      }
                      frame "右" {
                      }
                      frame "停" {
                      }
                    }
                  }
                }
                n220 = Build Array(u8 170 ("元素"), u8 175 ("元素"), u8 2 ("元素"), u8 1 ("元素"), w356) -> (w359:u8[])
                n221 = Add Array Elements(numeric array=w359) -> (sum=w358:u8)
                n222 = Build Array (concatenate)(w359, w358) -> (w357:u8[])
                n223 = Byte Array To String(unsigned byte array=w357) -> (string=w364:string)
                n224 = UDP Write(address=w354, port or service name=w355, connection ID=w353, data in=w364) -> ()  [unwired: 2 in, 2 out]
              }
              event "WRITE": Value Change {
                n225 = event-data() -> ()  [unwired: 1 in, 1 out]
                n226 = UDP Write(address=w377, port or service name=w376, connection ID=w378, data in="数据输入") -> ()  [unwired: 2 in, 2 out]
              }
              event "QUIT": Value Change {
                n227 = event-data() -> ()  [unwired: 1 in, 1 out]
                n228 = UDP Close(connection ID=w382) -> ()  [unwired: 1 in, 2 out]
                n229 = local read "主要"() -> (w379:refnum<k7>)
                n230 = local read "前摄像头"() -> (w381:refnum<k7>)
                n231 = local read "后摄像头"() -> (w380:refnum<k7>)
                n232 = invoke class="Web" method="StopRealPlayAll"(reference=w379) -> ()  [unwired: 2 in, 3 out]
                n233 = invoke class="Web" method="StopRealPlayAll"(reference=w381) -> ()  [unwired: 2 in, 3 out]
                n234 = invoke class="Web" method="StopRealPlayAll"(reference=w380) -> ()  [unwired: 2 in, 3 out]
              }
            }
          }
          frame #1 {
            n235 = local read "PITCH"() -> (w386:i32)
            n236 = local read "缩放"() -> (w408:dbl)
            n237 = local read "上下移动"() -> (w406:dbl)
            n238 = local read "前后移动"() -> (w405:dbl)
            n239 = Divide(x=w408, y=10.0) -> (x/y=w412:dbl)
            n240 = local read "左右移动"() -> (w407:dbl)
            n241 = Bundle By Name(cluster=cluster{"x":dbl, "y":dbl, "z":dbl} {"x"=0.0, "y"=0.0, "z"=0.0}, "x"=w412, "y"=w412, "z"=w412) -> (w385:cluster{"x":dbl, "y":dbl, "z":dbl})
            n242 = call <vilib>:"Clear Transformation.vi"("Object Refnum In"=w389) -> ("Object Refnum Out"=w384:refnum<vi>)  [unwired: 9 in, 1 out]
            n243 = local read "HEANDING"() -> (w387:i32)
            n244 = call <vilib>:"Scale Object.vi"("Scale"=w385, "Scene.Object In"=w384) -> ("Scene.Object Out"=w414:refnum<vi>)  [unwired: 8 in, 1 out]
            n245 = Bundle By Name(cluster=cluster{"x":dbl, "y":dbl, "z":dbl} {"x"=0.0, "y"=0.0, "z"=0.0}, "z"=w407, "y"=w406, "x"=w405) -> (w411:cluster{"x":dbl, "y":dbl, "z":dbl})
            n246 = Divide(x=w386, y=1000) -> (x/y=w392:dbl)
            n247 = local read "BANK"() -> (w388:i32)
            n248 = call <vilib>:"Set Translation.vi"("Translation"=w411, "Scene Object"=w414) -> ("Translated Object"=w402:refnum<vi>)  [unwired: 8 in, 1 out]
            n249 = Divide(x=w387, y=1000) -> (x/y=w393:dbl)
            n250 = call <vilib>:"Rotate X-axis.vi"("Relative?"=TRUE, "angle"=w392, "Scene Object In"=w402) -> ("error out"=w401:errorcluster, "Scene Object Out"=w400:refnum<vi>)  [unwired: 7 in]
            n251 = Divide(x=w388, y=1000) -> (x/y=w391:dbl)
            n252 = call <vilib>:"Rotate Z-axis.vi"("Relative?"=TRUE, "error in (no error)"=w401, "angle"=w393, "Scene Object In"=w400) -> ("error out"=w397:errorcluster, "Scene Object Out"=w396:refnum<vi>)  [unwired: 6 in]
            n253 = call <vilib>:"Rotate Y-axis.vi"("Relative?"=TRUE, "error in (no error)"=w397, "angle"=w391, "Scene Object In"=w396) -> ("Scene Object Out"=→"小车方向":refnum<vi>)  [unwired: 6 in, 1 out]
          }
        }
        n254 = Wait (ms)(milliseconds to wait=u32 100 ("等待时间（毫秒）")) -> ()  [unwired: 1 out]
      }
      frame Enabled {
      }
    }
  }
  n255 = flat-sequence {
    frame #0 {
      n256 = disable-structure shown="启用" {
        frame Disabled {
          n257 = invoke class="Web" method="Login"(reference="前摄像头", "lpServerIp"="192.168.0.28", "lPort"=34567, "lpUserName"="admin", "lpPassword"="") -> (reference out=w420:refnum<k7>, "Login"=→"Login":i32)  [unwired: 2 in, 5 out]
          n258 = invoke class="Web" method="StartChannelRealPlay"(reference=w420, "nChannel"=0, "lProtocolType"=0, "lStreamType"=0) -> ("StartChannelRealPlay"=→"后摄像头":bool)  [unwired: 2 in, 5 out]
        }
        frame Enabled {
        }
      }
    }
    frame #1 {
      n259 = Wait (ms)(milliseconds to wait=u32 10 ("等待时间（毫秒）")) -> ()  [unwired: 1 out]
    }
    frame #2 {
      n260 = disable-structure shown="禁用" {
        frame Disabled {
          n261 = invoke class="Web" method="Login"(reference="后摄像头", "lpServerIp"="192.168.0.108", "lPort"=34567, "lpUserName"="admin", "lpPassword"="") -> (reference out=w434:refnum<k7>, "Login"=→"Login 2":i32)  [unwired: 2 in, 5 out]
          n262 = invoke class="Web" method="StartChannelRealPlay"(reference=w434, "nChannel"=0, "lProtocolType"=0, "lStreamType"=0) -> ("StartChannelRealPlay"=→"前摄像头":bool)  [unwired: 2 in, 5 out]
        }
        frame Enabled {
        }
      }
    }
    frame #3 {
      n263 = Wait (ms)(milliseconds to wait=u32 10 ("等待时间（毫秒）")) -> ()  [unwired: 1 out]
    }
    frame #4 {
      n264 = disable-structure shown="禁用" {
        frame Disabled {
          n265 = flat-sequence {
            tunnel: [w442] -> w440
            tunnel: w440 -> [w447]
            frame #0 {
              n266 = invoke class="Web" method="Login"(reference="主要", "lpServerIp"="192.168.0.6", "lPort"=34567, "lpUserName"="admin", "lpPassword"="") -> (reference out=w442:refnum<k7>)  [unwired: 2 in, 6 out]
            }
            frame #1 {
              n267 = invoke class="Web" method="StartChannelRealPlay"(reference=w447, "nChannel"=0, "lProtocolType"=0, "lStreamType"=0) -> ()  [unwired: 2 in, 6 out]
              n268 = invoke class="Web" method="ChangeShowWndNum"(reference=w447, "nShowNum"=1, "bChangeOcx"=TRUE, "nSplit"=0, "nPreview"=1) -> ()  [unwired: 2 in, 7 out]
            }
          }
        }
        frame Enabled {
        }
      }
    }
  }
